vi "Update Test Step.vi"(8 "error in (no error)":errorcluster, 11 "TestExec in":refnum<class "TestExec.lvclass">) -> (0 "error out":errorcluster, 2 "Done?":bool, 3 "TestExec out":refnum<class "TestExec.lvclass">)   [LabVIEW 2019, in "Sequence Main.lvlib" / "TestExec.lvclass"]
uses:
  TestExec.lvclass
  TestExec.lvclass/TestExec.ctl
  <vilib>/addons/TestStand/_TSUtility.llb/TestStand - Get Property Value (Boolean Array).vi
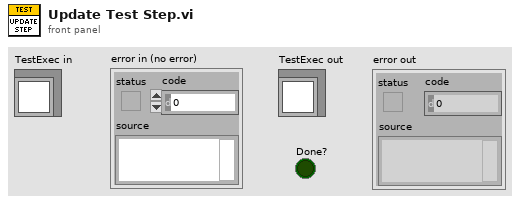
[diagram p1: front panel]
types:
  T1 = cluster{"Value[0]":bool, "Value[1]":bool, "Value[2]":bool, "Value[3]":bool, "Value[4]":bool, "Value[5]":bool, "Value[6]":bool}
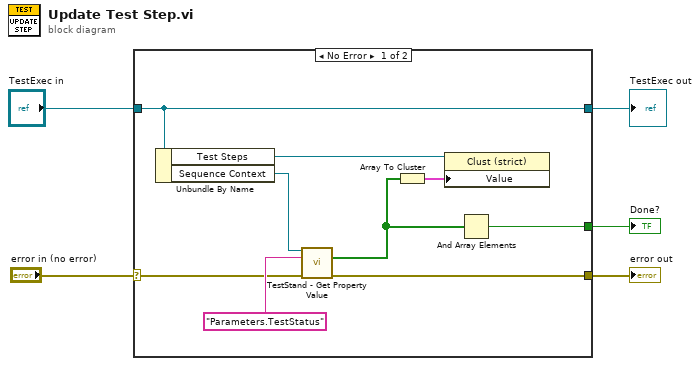
[diagram p0: block diagram]
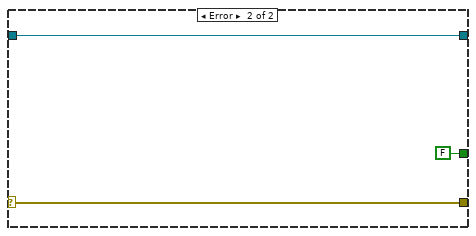
[diagram p2: hidden frame]
diagram:
  n1 = case shown="No Error" "error in (no error)" {
    selector: "error in (no error)" -> [w9 w17]
    tunnel: [w8 w17] -> w4
    tunnel: [w13 w16] -> w2
    tunnel: "TestExec in" -> [w13 w16]
    tunnel: [w6 FALSE] -> w1
    frame No Error {
      n2 = Unbundle By Name(w13) -> ("Test Steps"=w10:refnum<vi>, "Sequence Context"=w12:refnum<k7>)
      n3 = call-poly <vilib>:"TestStand - Get Property Value.vi"("Sequence Context In"=w12, "Lookup String"="Parameters.TestStatus", "error in (no error)"=w9) -> ("Value"=w7:bool[], "error out"=w8:errorcluster)  [unwired: 10 in, 1 out]
      n4 = Array To Cluster(array=w7) -> (cluster=w11:T1)
      n5 = property class="Clust (strict)"(reference=w10, "Value"=w11) -> ()  [unwired: 1 in, 2 out]
      n6 = And Array Elements(Boolean array=w7) -> (logical AND=w6:bool)
    }
    frame Error {
    }
  }
  "error out" <- w4
  "TestExec out" <- w2
  "Done?" <- w1
